vi "xps_panel_write_xps_panel_references.vi"(8 "error in (no error)":errorcluster, 10 "xps_panel_references":T1, 11 "newport_xps_panel in":refnum<class "newport_xps_panel.lvclass">) -> (0 "error out":errorcluster, 3 "newport_xps_panel out":refnum<class "newport_xps_panel.lvclass">)   [LabVIEW 2015, in "newport_xps_panel.lvclass"]
uses:
  newport_xps_panel.lvclass
  xps_panel_references.ctl
  newport_xps_panel.lvclass/newport_xps_panel.ctl
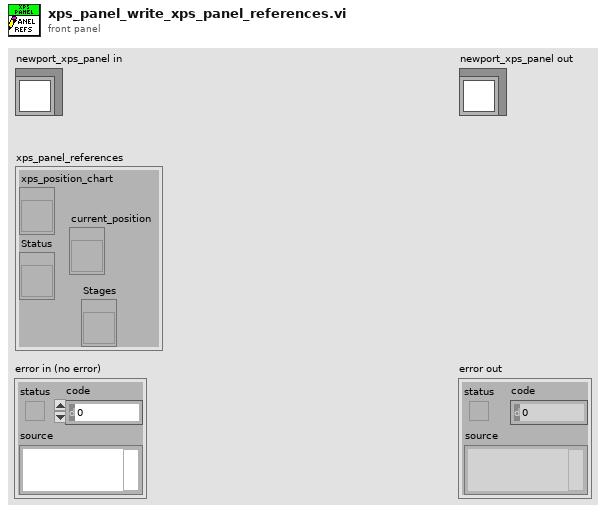
[diagram p1: front panel]
types:
  T1 = typedef "xps_panel_references.ctl" = cluster{"xps_position_chart":refnum<vi>, "Status":refnum<vi>, "current_position":refnum<vi>, "Stages":refnum<vi>}
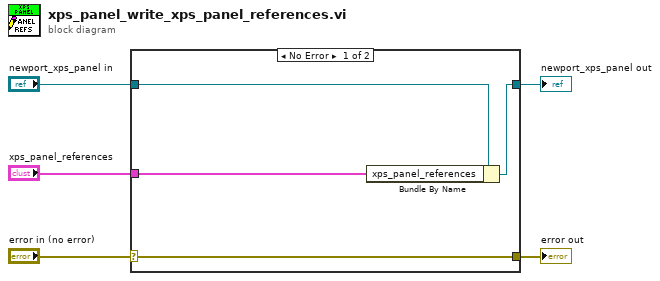
[diagram p0: block diagram]
diagram:
  n1 = case shown="No Error" "error in (no error)" {
    selector: "error in (no error)" -> [w9 w10]
    tunnel: [w9 w10] -> w4
    tunnel: [w7 w11] -> w2
    tunnel: "newport_xps_panel in" -> [w8 w11]
    tunnel: "xps_panel_references" -> [w6 _]
    frame No Error {
      n2 = Bundle By Name(cluster=w8, "xps_panel_references"=w6) -> (w7:refnum<class "newport_xps_panel.lvclass">)
    }
    frame Error {
    }
  }
  "error out" <- w4
  "newport_xps_panel out" <- w2
